vi "多参校准第三步.vi"(10 "标样1浓度输出":dbl, 11 "探头选择":u16(ring)=9 items=["氨氮"=3, "水温"=9, "pH值"=10, "溶解氧"=11, "电导率"=12, "浊度"=13, "叶绿素a"=14, "藻密度"=15, "蓝绿藻"=16, "氧化还原电位"=17, "溶解氧%"=18, "盐度"=19]) -> (2 "mean":dbl, 3 "继续执行":bool)   [LabVIEW 2016, in "斯坦道仪器.lvlib"]
uses:
  <vilib>/Analysis/NI_AALBase.lvlib
panel:
  out "B":dbl caption="校准值B:"
  out "K":dbl caption="校准值K:"
  out "x/y":dbl format="%#_6f"
  in  "测量数据区":i32(listbox)
  out "校准中":u8(slide) scale=0.0..180.0
  in  "取消":bool
  in  "校准确认":bool
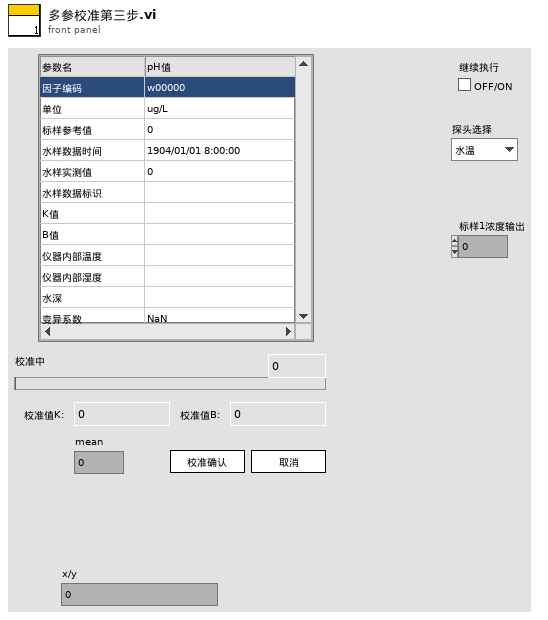
[diagram p1: front panel]
types:
  T1 = cluster{"因子编码":string, "单位":string, "标样参考值":sgl, "水样数据时间":timestamp, "水样实测值":sgl, "水样数据标识":string, "K":sgl, "B":sgl, "T":sgl, "H":sgl, "水深":sgl, "探头温度":sgl}
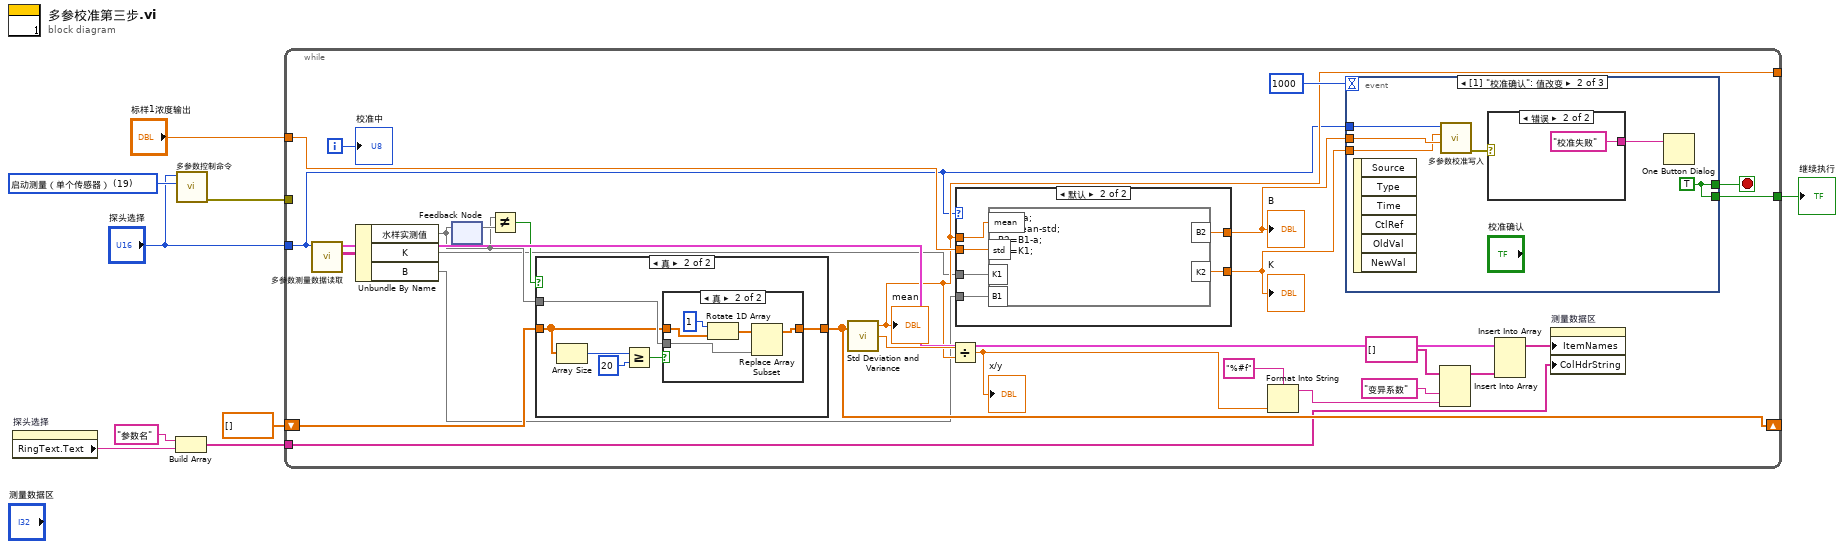
[diagram p0: block diagram]
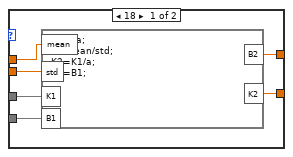
[diagram p2: hidden frame]
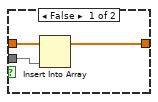
[diagram p4: hidden frame]
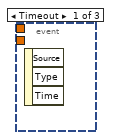
[diagram p5: hidden frame]
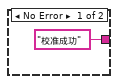
[diagram p6: hidden frame]
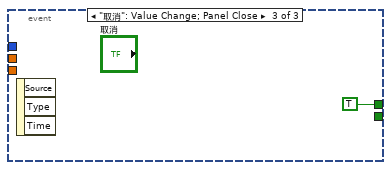
[diagram p7: hidden frame]
diagram:
  w7 = u16 19 items=["启动测量（全部）"=1, "初始化（清洗）"=10, "停止测量（全部）"=11, "校时"=13, "启动测量（单个传感器）"=19, "停止测量（单个传感器）"=20] ("控制命令")
  n1 = property on="探头选择" class="Ring (严格)"() -> ("RingText.Text"=w4:string)  [unwired: 2 in, 2 out]
  n2 = Build Array("参数名" ("元素"), w4) -> (w2:string[])
  n3 = call "多参数控制命令.vi"("控制命令"=w7, "站号"="探头选择") -> ("error out"=w6:errorcluster)  [unwired: 9 in]
  n4 = while {
    tunnel: [w36] -> w9
    shift-right: [w32] -> _
    shift-left: sgl[] [] ("数组") -> [w31]
    tunnel: "探头选择" -> [w14]
    tunnel: w6 -> [_]
    tunnel: [w17] -> _
    tunnel: w2 -> [w19]
    tunnel: "标样1浓度输出" -> [w18]
    i -> [w33]
    stop <- w35 stop-if-true
    n5 = call "多参数测量数据读取.vi"("探头选择"=w14) -> ("添加的数组"=w13:string[][], "测量数据块"=w27:T1)  [unwired: 8 in, 1 out]
    n6 = Unbundle By Name(w13) -> ("水样实测值"=w12, "K"=w11, "B"=w10)
    n7 = feedback-in #1(w12) -> ()
    n8 = feedback #1() -> (w21)  [unwired: 1 in]
    n9 = Not Equal?(x=w12, y=w21) -> (x != y?=w20:bool)
    n10 = case shown="真" w20 {
      tunnel: w12 -> [_ w55]
      tunnel: [w49 w54] -> w32
      tunnel: w31 -> [w49 w53]
      frame False {
      }
      frame True {
        n11 = Array Size(array=w53) -> (size(s)=w52:i32)
        n12 = Greater Or Equal?(x=w52, y=20) -> (x >= y?=w50:bool)
        n13 = case shown="真" w50 {
          tunnel: w55 -> [w58 w63]
          tunnel: [w57 w62] -> w54
          tunnel: w53 -> [w56 w61]
          frame False {
            n14 = Insert Into Array(array=w56, new element=w58) -> (w57:sgl[])  [unwired: 1 in]
          }
          frame True {
            n15 = Rotate 1D Array(1:w61, 2:1 ("n")) -> (0:w60:sgl[])
            n16 = Replace Array Subset(array=w60, new element=w63) -> (w62:sgl[])  [unwired: 1 in]
          }
        }
      }
    }
    n17 = call <vilib>:"Std Deviation and Variance.vi"("X"=w32) -> ("mean"=w17:dbl, "standard deviation"=w30:dbl)  [unwired: 1 in, 1 out]
    "mean" <- w17
    n18 = Divide(x=w30, y=w17) -> (x/y=w29:dbl)
    "x/y" <- w29
    n19 = case shown="默认" w14 {
      tunnel: w18 -> [w41 w48]
      tunnel: w10 -> [w39 w47]
      tunnel: [w38 w46] -> w15
      tunnel: w17 -> [w42 w45]
      tunnel: w11 -> [w40 w44]
      tunnel: [w37 w43] -> w16
      frame 18 {
        n20 = formula code="float a;\na=mean/std;\nK2=K1/a;\nB2=B1;"("mean"=w42, "std"=w41, "B1"=w39, "K1"=w40) -> ("B2"=w38:dbl, "K2"=w37:dbl)
      }
      frame Default {
        n21 = formula code="float a;\na=mean-std;\nB2=B1-a;\nK2=K1;"("mean"=w45, "std"=w48, "B1"=w47, "K1"=w44) -> ("B2"=w46:dbl, "K2"=w43:dbl)
      }
    }
    "B" <- w15
    "K" <- w16
    n22 = Format Into String(format string="%#f" ("格式字符串"), w29) -> (resulting string=w25:string)  [unwired: 2 in, 1 out]
    n23 = event shown="[1] \"校准确认\": 值改变" {
      selector: _ -> [_ _ _]
      dyn-events: _ -> [_ _ _]
      timeout: 1000 -> [_ _ _]
      tunnel: [_ w69 _] -> w36
      tunnel: [_ w69 TRUE ("继续执行")] -> w35
      tunnel: w16 -> [_ w64 _]
      tunnel: w15 -> [_ w65 _]
      tunnel: w14 -> [_ w68 _]
      event Timeout {
        n24 = event-data() -> ()  [unwired: 1 in, 3 out]
      }
      event "校准确认": Value Change {
        w69 = TRUE ("继续执行")
        n25 = event-data() -> ()  [unwired: 1 in, 6 out]
        n26 = call "多参数校准写入.vi"("B"=w65, "K"=w64, "站号"=w68) -> ("error out"=w67:errorcluster)  [unwired: 8 in]
        n27 = case shown="错误" w67 {
          tunnel: ["校准成功" ("消息") "校准失败" ("消息")] -> w66
          frame No Error {
          }
          frame Error {
          }
        }
        n28 = One Button Dialog(message=w66) -> ()  [unwired: 1 in, 1 out]
      }
      event "取消": Value Change; Panel Close {
        n29 = event-data() -> ()  [unwired: 1 in, 3 out]
      }
    }
    n30 = Insert Into Array(array=string[] [] ("数组"), new element #1="变异系数" ("格式字符串"), new element #2=w25) -> (w23:string[])  [unwired: 1 in]
    n31 = Insert Into Array(array=w27, new element=w23) -> (w22:string[])  [unwired: 2 in]
    n32 = property on="测量数据区" class="MCListbox (严格)"("ItemNames"=w22, "ColHdrString"=w19) -> ()  [unwired: 2 in, 2 out]
    "校准中" <- w33
  }
  "继续执行" <- w9
